vi "jitter.vi"() -> ()   [LabVIEW 2019]
uses:
  <vilib>/DAQmx/read.llb/DAQmx Read (Counter 1D DBL 1Chan NSamp).vi
  <vilib>/DAQmx/create/channels.llb/DAQmx Create Channel (CI-Period).vi
  <vilib>/DAQmx/configure/timing.llb/DAQmx Timing (Implicit).vi
  <vilib>/DAQmx/miscellaneous.llb/DAQmx Fill In Error Info.vi
  <vilib>/Utility/file.llb/Write Delimited Spreadsheet (DBL).vi
  <resource>/objmgr/daqmx.rc
panel:
  out "samples per channel":i32=1000
  out "TotalSampPerChanAcquired":dbl
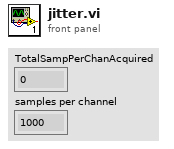
[diagram p1: front panel]
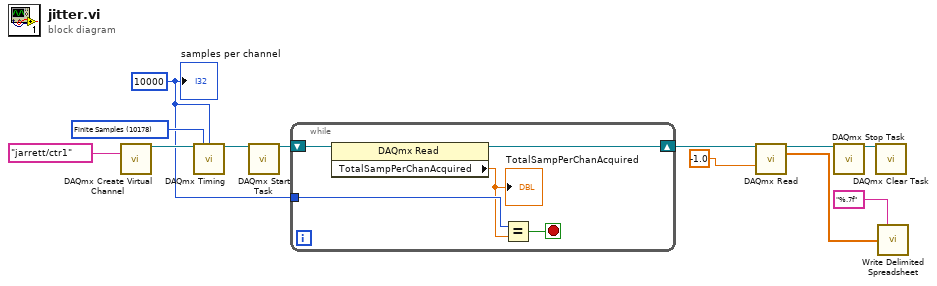
[diagram p0: block diagram]
diagram:
  w1 = 10000 ("samples per channel")
  w10 = 10178 items=["Finite Samples"=10178, "Continuous Samples"=10123, "Hardware Timed Single Point"=12522] ("sample mode")
  n1 = call-poly <vilib>:"DAQmx Create Virtual Channel.vi"("counter"=tag "jarrett/ctr1") -> ("task out"=w11:refnum<k21>)  [unwired: 13 in, 1 out]
  n2 = call-poly <vilib>:"DAQmx Timing.vi"("task/channels in"=w11, "sample mode"=w10, "samples per channel"=w1) -> ("task out"=w9:refnum<k21>)  [unwired: 11 in, 1 out]
  n3 = call <vilib>:"DAQmx Start Task.vi"("task/channels in"=w9) -> ("task out"=w3:refnum<k21>)  [unwired: 13 in, 1 out]
  n4 = while {
    tunnel: w1 -> [w15]
    shift-right: [w16] -> w2
    shift-left: w3 -> [w17]
    stop <- w13 stop-if-true
    n5 = property class="DAQmx Read"(reference=w17) -> (reference out=w16:refnum<k21>, "TotalSampPerChanAcquired"=w14:dbl)  [unwired: 1 in, 1 out]
    "TotalSampPerChanAcquired" <- w14
    n6 = Equal?(x=w15, y=w14) -> (x = y?=w13:bool)
  }
  n7 = call-poly <vilib>:"DAQmx Read.vi"("task/channels in"=w2, "timeout"=-1.0) -> ("task out"=w8:refnum<k21>, "data"=w5:dbl[])  [unwired: 11 in, 1 out]
  n8 = call <vilib>:"DAQmx Stop Task.vi"("task/channels in"=w8) -> ("task out"=w7:refnum<k21>)  [unwired: 13 in, 1 out]
  n9 = call <vilib>:"DAQmx Clear Task.vi"("task in"=w7) -> ()  [unwired: 14 in, 1 out]
  n10 = call-poly <vilib>:"Write Delimited Spreadsheet.vi"("format (%.3f)"="%.7f", "1D data"=w5) -> ()  [unwired: 12 in, 2 out]
  "samples per channel" <- w1
